vi "Symmetrical Components (1 Cycle).vi"(0 "one-cycle fundamental voltage vectors":T3(array[cluster]), 5 "one-cycle fundamental current vectors":T3(array[cluster]), 9 "system info in":refnum<class "EP System Info.lvclass">, 11 "error in (no error)":errorcluster) -> (4 "one-cycle fundamental symmetrical components":T1(array[cluster]), 10 "system info out":refnum<class "EP System Info.lvclass">, 15 "error out":errorcluster)   [LabVIEW 2014, in "NI_EP_Power Quality.lvlib"]
doc: "Calculates the fundamental voltage, current, and power symmetrical components for a single-cycle block.\n\nThis VI supports measuring single-line and multiple-line systems."
uses:
  <vilib>/addons/Electrical Power/PQ/NI_EP_Power Quality.lvlib
  <vilib>/addons/Electrical Power/PQ/Common/Controls/ep_AI Data Channel.ctl
  <vilib>/addons/Electrical Power/PQ/Common/Classes/System Info/EP System Info.lvclass
  <vilib>/addons/Electrical Power/Motor Monitoring/NI_EP_Motor Monitoring.lvlib
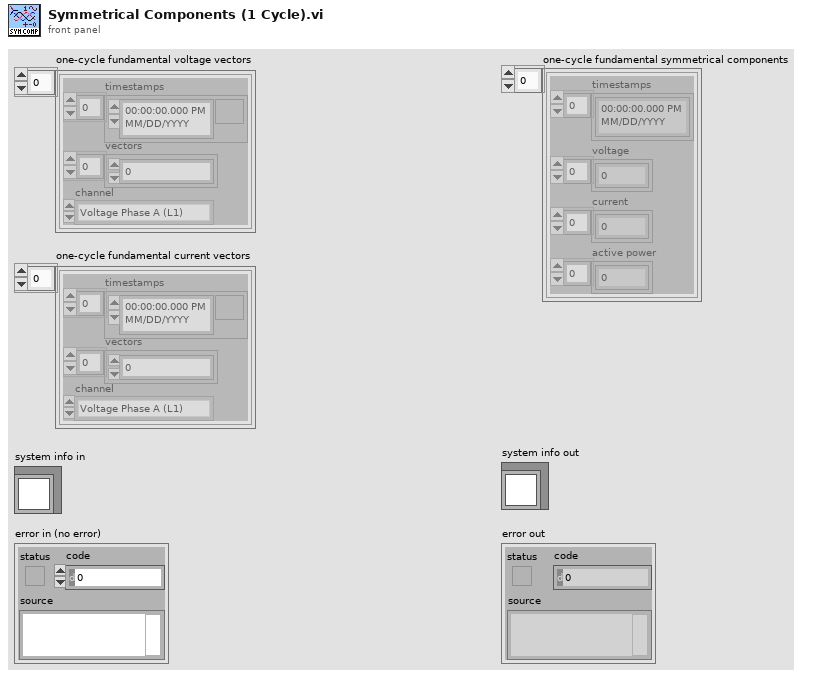
[diagram p1: front panel]
types:
  T1 = cluster{"timestamps":timestamp[], "voltage":dbl[], "current":dbl[], "active power":dbl[]}[]
  T2 = typedef "NI_EP_Power Quality.lvlib/ep_AI Data Channel.ctl" = enum16{"Voltage Phase A (L1)", "Voltage Phase B (L2)", "Voltage Phase C (L3)", "Voltage Phase N (Neutral)", "Current Phase A (L1)", "Current Phase B (L2)", "Current Phase C (L3)", "Current Phase N (Neutral)"}
  T3 = cluster{"timestamps":timestamp[], "vectors":cdb[], "channel":T2}[]
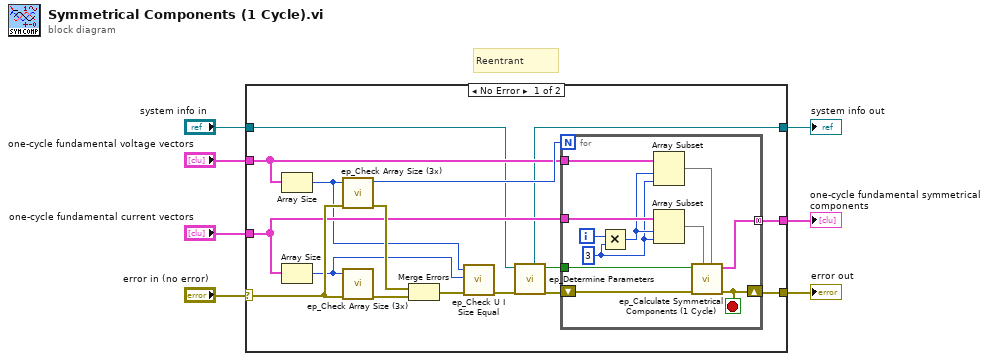
[diagram p0: block diagram]
diagram:
  # "Reentrant"
  n1 = case shown="No Error" "error in (no error)" {
    selector: "error in (no error)" -> [w21 w35]
    tunnel: "system info in" -> [w14 w36]
    tunnel: "one-cycle fundamental voltage vectors" -> [w16 _]
    tunnel: "one-cycle fundamental current vectors" -> [w15 _]
    tunnel: [w23 w35] -> w4
    tunnel: [w13 w36] -> w3
    tunnel: [w18 _] -> w1
    frame No Error {
      n2 = Array Size(array=w16) -> (size(s)=w10:i32)
      n3 = Array Size(array=w15) -> (size(s)=w9:i32)
      n4 = call <vilib>:"ep_Check Array Size (3x).vi"("error in (no error)"=w21, "number of channels"=w10) -> ("error out"=w20:errorcluster, "number of 3 phases"=w17:i32)  [unwired: 8 in]
      n5 = call <vilib>:"ep_Check Array Size (3x).vi"("error in (no error)"=w21, "number of channels"=w9) -> ("error out"=w19:errorcluster)  [unwired: 8 in, 1 out]
      n6 = Merge Errors(w20, w19) -> (w12:errorcluster)
      n7 = call <vilib>:"ep_Check U I Size Equal.vi"("error in (no error)"=w12, "current channel number"=w9, "voltage channel number"=w10) -> ("error out"=w11:errorcluster)  [unwired: 8 in]
      n8 = call <vilib>:"ep_Determine Parameters.vi"("error in (no error)"=w11, "system info in"=w14) -> ("error out"=w22:errorcluster, "line voltage?"=w8:bool, "system info out"=w13:refnum<class "EP System Info.lvclass">)  [unwired: 6 in, 1 out]
      n9 = for {
        N: w17 -> [_]
        shift-right: [w33] -> w23
        shift-left: w22 -> [w34]
        tunnel: [w32] -> w18 mode=concatenating
        tunnel: w16 -> [w30]
        tunnel: w15 -> [w28]
        tunnel: w8 -> [w24]
        i -> [w27]
        stop <- w33 stop-if-true
        w25 = 3 ("y")
        n10 = Multiply(x=w27, y=w25) -> (x*y=w26:i32)
        n11 = Array Subset(array=w30, index=w26, length=w25) -> (w31:T3)
        n12 = Array Subset(array=w28, index=w26, length=w25) -> (w29:T3)
        n13 = call <vilib>:"ep_Calculate Symmetrical Components (1 Cycle).vi"("one period fundamental voltage vectors"=w31, "one period fundamental current vectors"=w29, "error in (no error)"=w34, "line voltage? (F)"=w24) -> ("error out"=w33:errorcluster, "one-cycle fundamental symmetrical components"=w32:T1)  [unwired: 6 in]
      }
    }
    frame Error {
    }
  }
  "error out" <- w4
  "system info out" <- w3
  "one-cycle fundamental symmetrical components" <- w1
